vi "AVI U16 write-read.vi"() -> ()   [LabVIEW 2017]
doc: "This is a complete example on how to generate an AVI file from a set of 16bit (U16 or lower resolution) images/frames and read them back from the AVI file. Note that this will not work if you feed U32 data to the ArrayToColorImage vi."
panel:
  in  "U16 Image data (demo data)":u16[][](array[numeric])=array512x512[262144 elements]
  out "U16 Image":T1(plugin-control)
  out "OK":bool
  out "Data read back (U16)":u16[][][](array[numeric])
  out "RGB Image":T1(plugin-control)
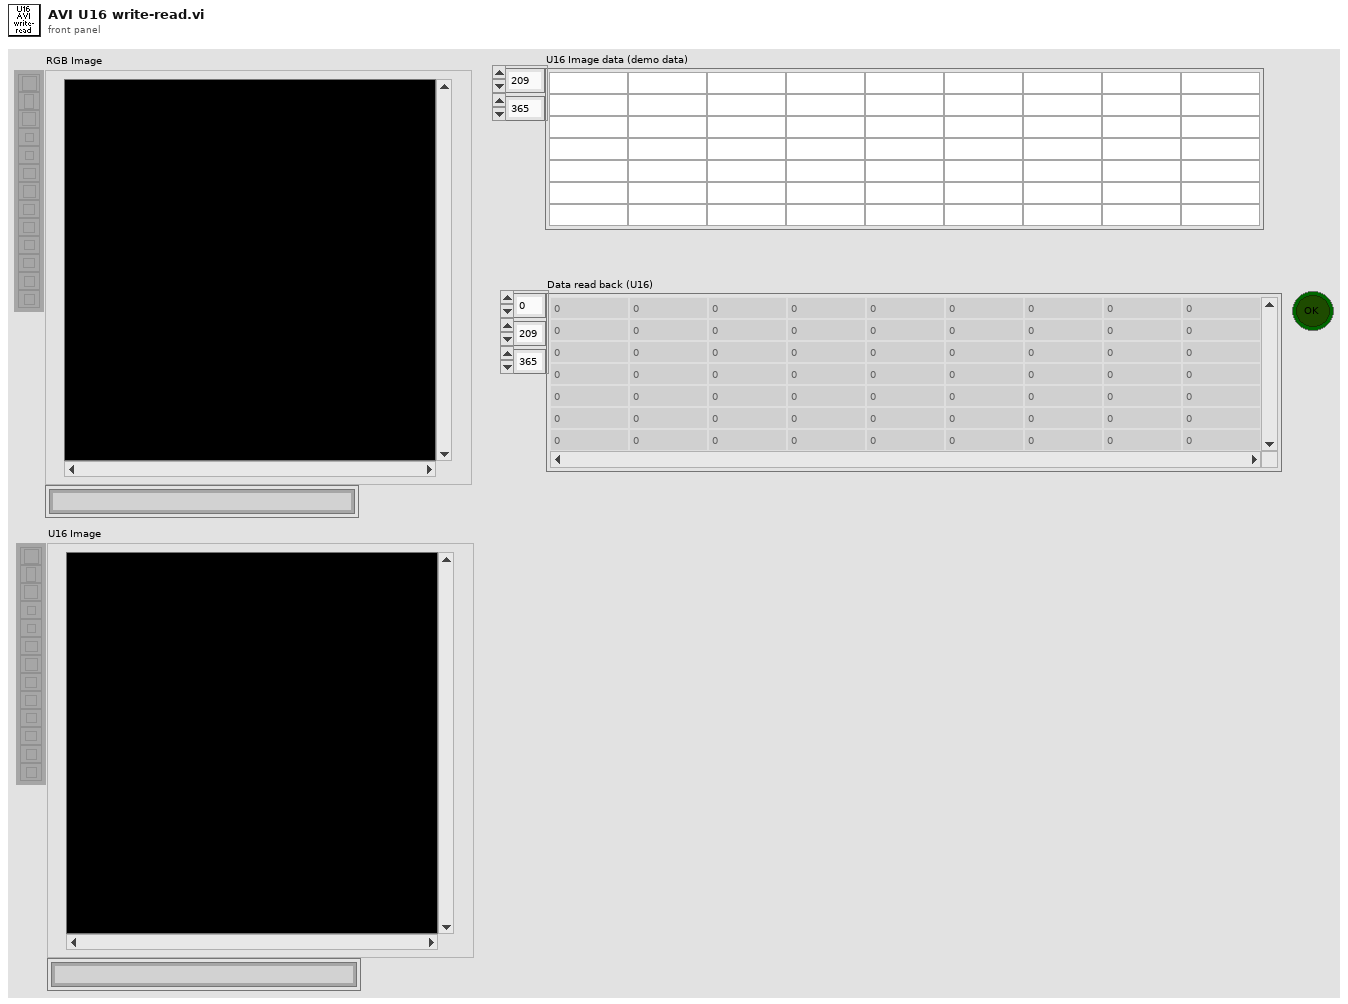
[diagram p1: front panel]
types:
  T1 = typedef "IMAQ Image.ctl" = refnum<image>
  T2 = typedef "Image Type" = u32
  T3 = typedef "AviRefnum.ctl" = refnum<k1>
  T4 = typedef "IMAQ AVI2 Refnum.ctl" = refnum<k20>
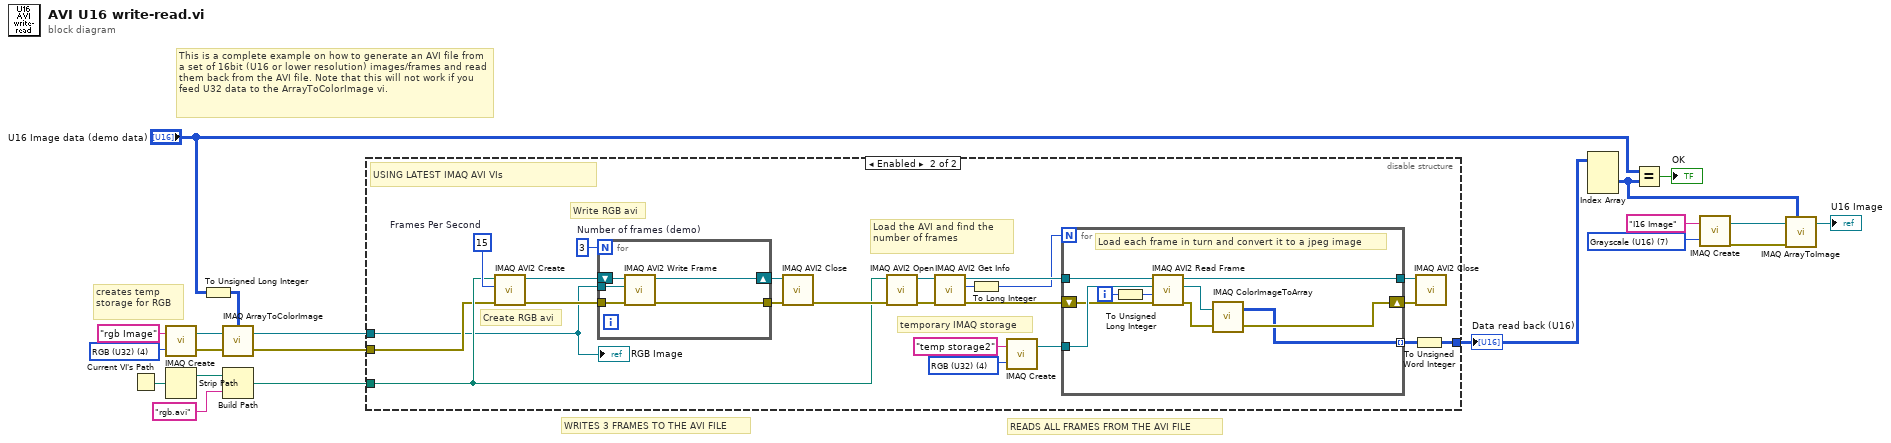
[diagram p0: block diagram]
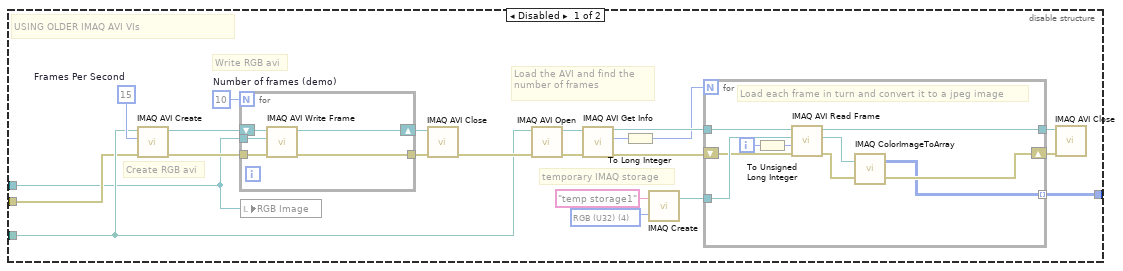
[diagram p2: hidden frame]
diagram:
  w8 = T2 7 items=["Grayscale (U8)", "Grayscale (I16)", "Grayscale (SGL)", "Complex (CSG)", "RGB (U32)", "HSL (U32)", "RGB (U64)", "Grayscale (U16)"] ("Image Type")
  w17 = T2 4 items=["Grayscale (U8)", "Grayscale (I16)", "Grayscale (SGL)", "Complex (CSG)", "RGB (U32)", "HSL (U32)", "RGB (U64)", "Grayscale (U16)"] ("Image Type")
  # "This is a complete example on how to generate an AVI file from a set of 16bit (U16 or lower resolution) images/frames and read them back from the AVI file. Note that this will not work if you feed U32 data to the ArrayToColorImage vi."
  # "WRITES 3 FRAMES TO THE AVI FILE"
  # "READS ALL FRAMES FROM THE AVI FILE"
  # "creates temp storage for RGB"
  n1 = Current VI's Path() -> (path=w20:path)
  n2 = call "IMAQ Create"("Image Name"="rgb Image", "Image Type"=w17) -> ("New Image"=w3:T1, "error out"=w15:errorcluster)  [unwired: 2 in, 1 out]
  n3 = Strip Path(path=w20) -> (stripped path=w19:path)  [unwired: 1 out]
  n4 = To Unsigned Long Integer(number="U16 Image data (demo data)") -> (unsigned 32bit integer=w2:u32[][])
  n5 = call "IMAQ ArrayToColorImage"("Image Pixels (U32)"=w2, "Image"=w3, "error in (no error)"=w15) -> ("Image Out"=w10:T1, "error out"=w11:errorcluster)  [unwired: 1 in, 1 out]
  n6 = Build Path(base path=w19, name or relative path="rgb.avi") -> (appended path=w14:path)
  n7 = disable-structure shown="Enabled" {
    disable-tunnel: w14 -> [w25 w61]
    disable-tunnel: [w24 w59] -> w13
    disable-tunnel: w11 -> [w23 w60]
    disable-tunnel: w10 -> [w21 w58]
    frame Disabled {
      w32 = T2 4 items=["Grayscale (U8)", "Grayscale (I16)", "Grayscale (SGL)", "Complex (CSG)", "RGB (U32)", "HSL (U32)", "RGB (U64)", "Grayscale (U16)"] ("Image Type")
      w38 = 10  # Number of frames (demo)
      w37 = u32 15  # Frames Per Second
      # "USING OLDER IMAQ AVI VIs"
      # "temporary IMAQ storage"
      # "Load the AVI and find the number of frames"
      # "Write RGB avi"
      # "Create RGB avi"
      n8 = call "IMAQ AVI Create"("error in (no error)"=w23, "Frames Per Second"=w37, "AVI Path"=w25) -> ("error out"=w41:errorcluster, "Avi Refnum"=w39:T3)  [unwired: 4 in, 3 out]
      n9 = for {
        N: w38 -> [_]
        shift-right: [w56] -> w40
        shift-left: w39 -> [w57]
        tunnel: w21 -> [w55]
        tunnel: w41 -> [w54]
        tunnel: [w53] -> w42
        n10 = call "IMAQ AVI Write Frame"("error in (no error)"=w54, "Image"=w55, "Avi Refnum"=w57) -> ("error out"=w53:errorcluster, "Avi Refnum (duplicate)"=w56:T3)  [unwired: 1 in, 6 out]
      }
      n11 = local write "RGB Image"(w21) -> ()
      n12 = call "IMAQ AVI Close"("error in (no error)"=w42, "Avi Refnum"=w40) -> ("error out"=w26:errorcluster)  [unwired: 9 out]
      n13 = call "IMAQ AVI Open"("error in (no error)"=w26, "AVI Path"=w25) -> ("error out"=w33:errorcluster, "Avi Refnum"=w28:T3)  [unwired: 8 out]
      n14 = call "IMAQ AVI Get Info"("error in (no error)"=w33, "Avi Refnum"=w28) -> ("error out"=w34:errorcluster, "Number of Frames"=w36:u32, "Avi Refnum (duplicate)"=w30:T3)  [unwired: 7 out]
      n15 = To Long Integer(number=w36) -> (32bit integer=w22:i32)
      n16 = call "IMAQ Create"("Image Name"="temp storage1", "Image Type"=w32) -> ("New Image"=w27:T1)  [unwired: 2 in, 2 out]
      n17 = for {
        N: w22 -> [_]
        tunnel: w27 -> [w51]
        tunnel: [w50] -> w29
        tunnel: w30 -> [w49]
        shift-right: [w45] -> w35
        shift-left: w34 -> [w48]
        tunnel: [w44] -> w24 mode=indexing
        i -> [w47]
        # "Load each frame in turn and convert it to a jpeg image"
        n18 = To Unsigned Long Integer(number=w47) -> (unsigned 32bit integer=w43:u32)
        n19 = call "IMAQ AVI Read Frame"("error in (no error)"=w48, "Frame Number"=w43, "Image"=w51, "Avi Refnum"=w49) -> ("error out"=w46:errorcluster, "Image Out"=w52:T1, "Avi Refnum (duplicate)"=w50:T3)  [unwired: 1 in, 4 out]
        n20 = call "IMAQ ColorImageToArray"("Image"=w52, "error in (no error)"=w46) -> ("Image Pixels (U32)"=w44:u32[][], "error out"=w45:errorcluster)  [unwired: 1 in, 2 out]
      }
      n21 = call "IMAQ AVI Close"("error in (no error)"=w35, "Avi Refnum"=w29) -> ()  [unwired: 10 out]
    }
    frame Enabled {
      w72 = T2 4 items=["Grayscale (U8)", "Grayscale (I16)", "Grayscale (SGL)", "Complex (CSG)", "RGB (U32)", "HSL (U32)", "RGB (U64)", "Grayscale (U16)"] ("Image Type")
      w63 = 3  # Number of frames (demo)
      w64 = u32 15  # Frames Per Second
      # "USING LATEST IMAQ AVI VIs"
      # "temporary IMAQ storage"
      # "Load the AVI and find the number of frames"
      # "Write RGB avi"
      # "Create RGB avi"
      n22 = call "IMAQ AVI2 Create"("error in (no error)"=w60, "Frames Per Second"=w64, "AVI Path"=w61) -> ("error out"=w65:errorcluster, "AVI Refnum"=w66:T4)  [unwired: 7 in]
      n23 = for {
        N: w63 -> [_]
        shift-right: [w93] -> w67
        shift-left: w66 -> [w95]
        tunnel: w58 -> [w94]
        tunnel: w65 -> [w91]
        tunnel: [w92] -> w68
        n24 = call "IMAQ AVI2 Write Frame"("error in (no error)"=w91, "Image"=w94, "AVI Refnum"=w95) -> ("error out"=w92:errorcluster, "AVI Refnum (duplicate)"=w93:T4)  [unwired: 6 in, 1 out]
      }
      n25 = call "IMAQ AVI2 Close"("error in (no error)"=w68, "AVI Refnum"=w67) -> ("error out"=w69:errorcluster)  [unwired: 9 in]
      n26 = call "IMAQ AVI2 Open"("error in (no error)"=w69, "AVI File Path"=w61) -> ("error out"=w73:errorcluster, "AVI Refnum"=w74:T4)  [unwired: 8 in]
      n27 = call "IMAQ AVI2 Get Info"("error in (no error)"=w73, "AVI Refnum"=w74) -> ("error out"=w76:errorcluster, "Number of Frames"=w75:u32, "AVI Refnum (duplicate)"=w78:T4)  [unwired: 5 in, 2 out]
      n28 = To Long Integer(number=w75) -> (32bit integer=w77:i32)
      n29 = call "IMAQ Create"("Image Name"="temp storage2", "Image Type"=w72) -> ("New Image"=w70:T1)  [unwired: 2 in, 2 out]
      n30 = for {
        N: w77 -> [_]
        tunnel: w70 -> [w85]
        tunnel: [w86] -> w79
        tunnel: w78 -> [w87]
        shift-right: [w89] -> w80
        shift-left: w76 -> [w82]
        tunnel: [w88] -> w62 mode=indexing
        i -> [w90]
        # "Load each frame in turn and convert it to a jpeg image"
        n31 = To Unsigned Long Integer(number=w90) -> (unsigned 32bit integer=w81:u32)
        n32 = call "IMAQ AVI2 Read Frame"("error in (no error)"=w82, "Frame Number"=w81, "Image"=w85, "AVI Refnum"=w87) -> ("error out"=w83:errorcluster, "Image Out"=w84:T1, "AVI Refnum (duplicate)"=w86:T4)  [unwired: 5 in]
        n33 = call "IMAQ ColorImageToArray"("Image"=w84, "error in (no error)"=w83) -> ("Image Pixels (U32)"=w88:u32[][], "error out"=w89:errorcluster)  [unwired: 1 in, 2 out]
      }
      n34 = To Unsigned Word Integer(number=w62) -> (unsigned 16bit integer=w59:u16[][][])
      n35 = call "IMAQ AVI2 Close"("error in (no error)"=w80, "AVI Refnum"=w79) -> ()  [unwired: 9 in, 1 out]
      "RGB Image" <- w58
    }
  }
  "Data read back (U16)" <- w13
  n36 = Index Array(array=w13) -> (element=w1:u16[][])  [unwired: 3 in]
  n37 = Equal?(x="U16 Image data (demo data)", y=w1) -> (x = y?=→"OK":bool)
  n38 = call "IMAQ Create"("Image Name"="I16 Image", "Image Type"=w8) -> ("New Image"=w7:T1, "error out"=w6:errorcluster)  [unwired: 2 in, 1 out]
  n39 = call "IMAQ ArrayToImage"("Image Pixels (U16)"=w1, "error in (no error)"=w6, "Image"=w7) -> ("Image Out"=→"U16 Image":T1)  [unwired: 7 in, 1 out]
